vi "Utility Check for Error Response.vi"(10 "error in (no error)":errorcluster, 11 "Response String (in)":string) -> (2 "error out":errorcluster, 3 "Response String (out)":string)   [LabVIEW 2020, in "Omega Platinum Series.lvlib"]
doc: "Checks for an error response message. If one is found, a custom error cluster is created with Status = True and Code = 6000 for an Invalid Command. The response string is returned without alteration for use down the data wire."
uses:
  Omega Platinum Series.lvlib
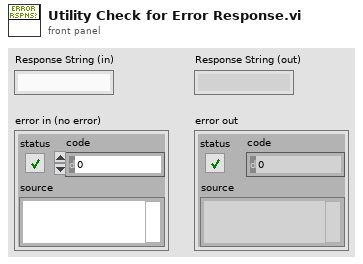
[diagram p1: front panel]
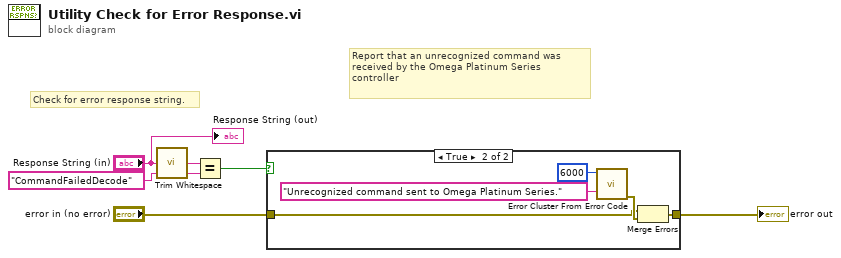
[diagram p0: block diagram]
diagram:
  # "Report that an unrecognized command was received by the Omega Platinum Series controller"
  # "Check for error response string."
  n1 = call <vilib>:"Trim Whitespace.vi"("string"="Response String (in)") -> ("trimmed string"=w4:string)  [unwired: 1 in]
  n2 = Equal?(x=w4, y="CommandFailedDecode") -> (x = y?=w3:bool)
  n3 = case shown="True" w3 {
    tunnel: [w7 w10] -> w1
    tunnel: "error in (no error)" -> [w7 w8]
    frame False {
    }
    frame True {
      n4 = call <vilib>:"Error Cluster From Error Code.vi"("error message (\"\")"="Unrecognized command sent to Omega Platinum Series." ("error message (\"\")"), "error code (0)"=6000) -> ("error out"=w9:errorcluster)  [unwired: 7 in]
      n5 = Merge Errors(w8, w9) -> (w10:errorcluster)
    }
  }
  "error out" <- w1
  "Response String (out)" <- "Response String (in)"
